vi "Recursive VI.vi"(11 "Number":dbl) -> (1 "Number to search":dbl, 2 "Match?":bool)   [LabVIEW 2023]
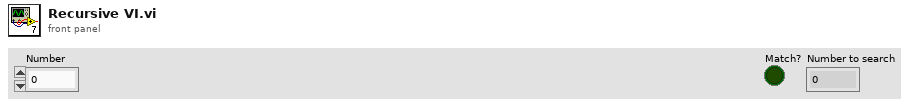
[diagram p1: front panel]
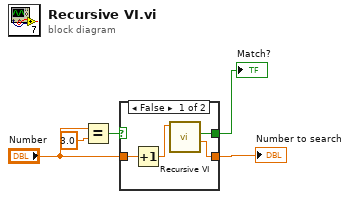
[diagram p0: block diagram]
diagram:
  n1 = Equal?(x="Number", y=3.0) -> (x = y?=w4:bool)
  n2 = case shown="False" w4 {
    selector: w4 -> [_ w10]
    tunnel: "Number" -> [w9 w11]
    tunnel: [w8 w10] -> w2
    tunnel: [w6 w11] -> w1
    frame False {
      n3 = Increment(x=w9) -> (x+1=w7:dbl)
      n4 = call "Recursive VI.vi"("Number"=w7) -> ("Number to search"=w6:dbl, "Match?"=w8:bool)  [unwired: 9 in]
    }
    frame True {
    }
  }
  "Match?" <- w2
  "Number to search" <- w1
